vi "OolingMilkTea_Create.vi"(8 "Error In":errorcluster, 11 "reference in":refnum<class "OolingMilkTea.lvclass">) -> (0 "Error Out":errorcluster, 3 "reference out":refnum<class "OolingMilkTea.lvclass">)   [LabVIEW 2020, in "OolingMilkTea.lvclass"]
uses:
  OolingMilkTea.lvclass
  Console_class/Console.lvclass
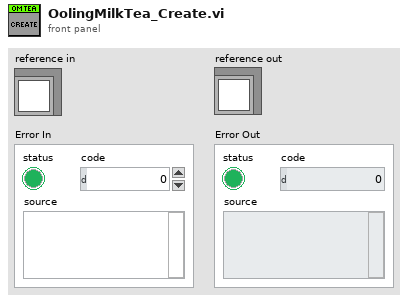
[diagram p1: front panel]
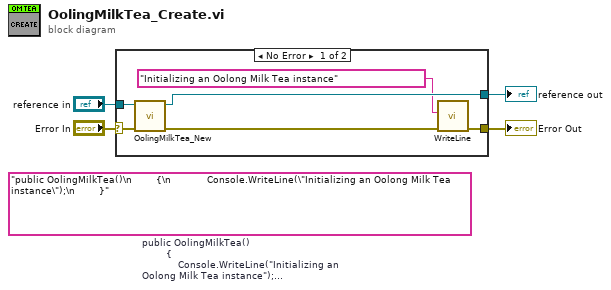
[diagram p0: block diagram]
diagram:
  (unwired) "public OolingMilkTea()\n        {\n            Console.WriteLine(\"Initializing an Oolong Milk Tea instance\");\n        }"  # public OolingMilkTea()         {             Console.WriteLine("Initializing an Oolong Milk Tea instance");         }
  n1 = case shown="No Error" "Error In" {
    selector: "Error In" -> [w9 w12]
    tunnel: [w6 w12] -> w3
    tunnel: "reference in" -> [w10 w11]
    tunnel: [w8 w11] -> w1
    frame No Error {
      n2 = call "OolingMilkTea_New.vi"("error in (no error)"=w9, "reference in"=w10) -> ("error out"=w7:errorcluster, "reference out"=w8:refnum<class "OolingMilkTea.lvclass">)  [unwired: 6 in, 2 out]
      n3 = call "WriteLine.vi"("Error In"=w7, "ConsoleText"="Initializing an Oolong Milk Tea instance") -> ("Error Out"=w6:errorcluster)  [unwired: 9 in]
    }
    frame Error {
      # "VI-TechBaseTemplate_Simple_4x4x4"
    }
  }
  "Error Out" <- w3
  "reference out" <- w1
